vi "Coerce Line Rate.vi"(9 "Line rate IN":dbl, 11 "Pixel format":T1 items=["Mono8"=257, "Mono10"=258, "Mono12"=259]) -> (1 "Line rate OUT":dbl)   [LabVIEW 2020]
uses:
  VPD Controls/VPD Pixel format.ctl
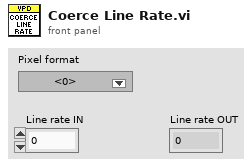
[diagram p1: front panel]
types:
  T1 = typedef "VPD Pixel format.ctl" = i64
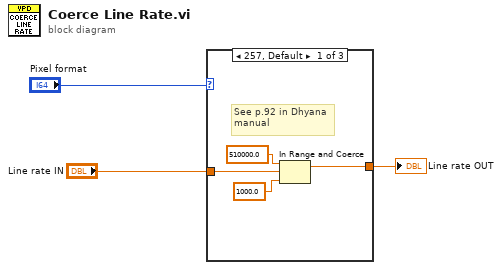
[diagram p0: block diagram]
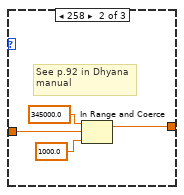
[diagram p2: hidden frame]
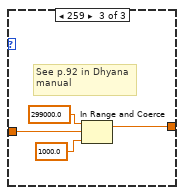
[diagram p3: hidden frame]
diagram:
  n1 = case shown="257, Default" "Pixel format" {
    tunnel: "Line rate IN" -> [w7 w11 w15]
    tunnel: [w4 w8 w12] -> w2
    frame 257, Default {
      # "See p.92 in Dhyana\nmanual"
      n2 = In Range and Coerce(upper limit=510000.0, x=w7, lower limit=1000.0) -> (coerced(x)=w4:dbl)  [unwired: 1 out]
    }
    frame 258 {
      # "See p.92 in Dhyana\nmanual"
      n3 = In Range and Coerce(upper limit=345000.0, x=w11, lower limit=1000.0) -> (coerced(x)=w8:dbl)  [unwired: 1 out]
    }
    frame 259 {
      # "See p.92 in Dhyana\nmanual"
      n4 = In Range and Coerce(upper limit=299000.0, x=w15, lower limit=1000.0) -> (coerced(x)=w12:dbl)  [unwired: 1 out]
    }
  }
  "Line rate OUT" <- w2
